vi "getTaskByName.vi"(10 "Task Name":string, 11 "BuildWorker in":refnum<class "BuildWorker.lvclass">) -> (1 "index of element":i32, 2 "Task":refnum<class "Task.lvclass">, 3 "BuildWorker out":refnum<class "BuildWorker.lvclass">)   [LabVIEW 2017, in "BuildWorker.lvlib" / "BuildWorker.lvclass"]
uses:
  BuildWorker.lvclass
  Classes/Task Interface/Task/Task.lvclass
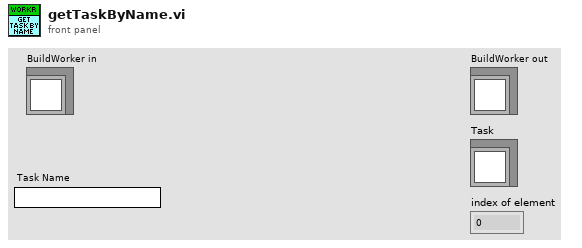
[diagram p1: front panel]
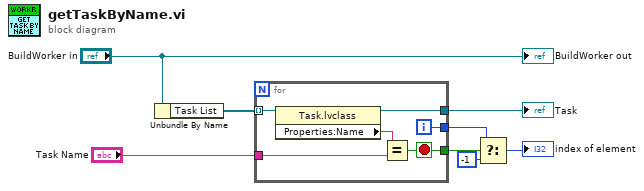
[diagram p0: block diagram]
diagram:
  n1 = Unbundle By Name("BuildWorker in") -> ("Task List"=w6:refnum<class "Task.lvclass">[])
  n2 = for {
    tunnel: w6 -> [w14] mode=indexing
    tunnel: "Task Name" -> [w12]
    tunnel: [w11] -> w5
    tunnel: [w10] -> w4
    tunnel: [w9] -> w1
    i -> [w10]
    stop <- w11 stop-if-true
    n3 = property class="Task.lvclass"(reference=w14) -> (reference out=w9:refnum<class "Task.lvclass">, "Properties:Name"=w13:string)  [unwired: 1 in, 1 out]
    n4 = Equal?(x=w13, y=w12) -> (x = y?=w11:bool)
  }
  "Task" <- w1
  n5 = Select(t=w4, s=w5, f=-1) -> (s? t:f=→"index of element":i32)
  "BuildWorker out" <- "BuildWorker in"
